vi "CSC_QuadPlannerLoose.vi"(5 "TorqueError(0)":T1, 6 "F range":cluster{"Fmin":dbl, "Fmax":dbl}, 7 "TargetF(N) (0)":dbl format="%#_13g", 8 "error in (no error)":errorcluster, 9 "LockedJoint":i32[](array[numeric]), 10 "DesireTorque(Nm)":dbl[](array[numeric]), 11 "C-Alex in":refnum<class "CableSerialChain.lvclass">) -> (0 "error out":errorcluster, 1 "Jacobian for Cables":T2, 2 "Planned Tension":dbl[](array[numeric]), 3 "C-Alex out":refnum<class "CableSerialChain.lvclass">, 4 "Solved":bool)   [LabVIEW 2015, in "CableSerialChain.lvclass"]
uses:
  CableSerialChain.lvclass
  <vilib>/Analysis/Matrix/Datatypes/RealMatrix.ctl
  <vilib>/gmath/NumericalOptimization/stopping criteria.ctl
  CableSerialChain.lvclass/CableSerialChain.ctl
  <vilib>/Analysis/7linalg.llb/Create Special Real Matrix.vi
  <vilib>/Analysis/Matrix/Numeric/Conversions/Matrix To Array - RM.vi
  <vilib>/gmath/NumericalOptimization/Quadratic Programming AS.vi
  <vilib>/gmath/NI_Gmath.lvlib
  <vilib>/Analysis/NI_AALPro.lvlib
  <vilib>/Analysis/Matrix/NI_Matrix.lvlib
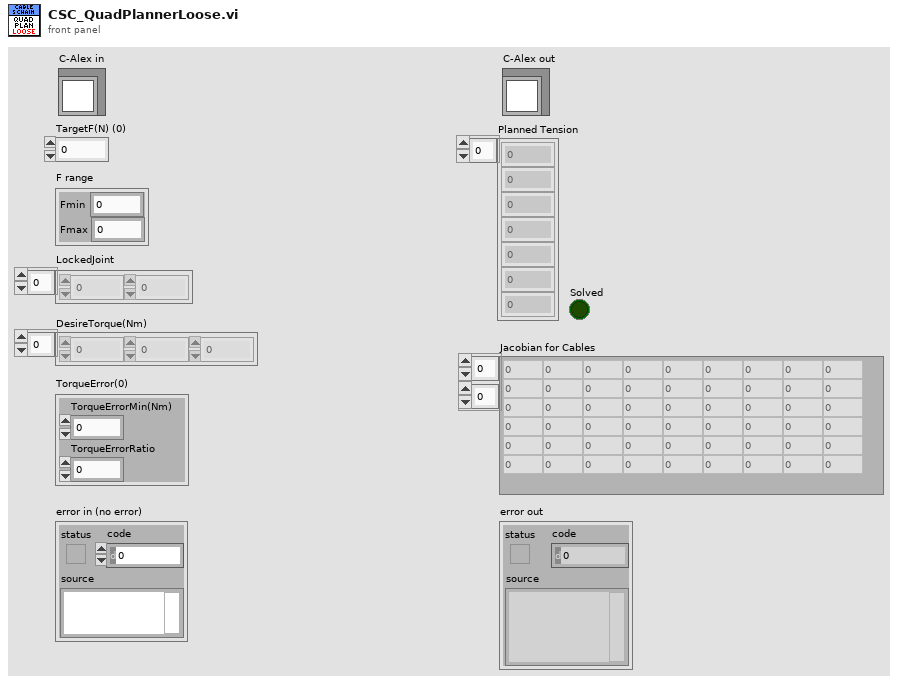
[diagram p1: front panel]
types:
  T1 = cluster{"TorqueErrorMin(Nm)":dbl, "TorqueErrorRatio":dbl}
  T2 = typedef "NI_Matrix.lvlib/RealMatrix.ctl" = dbl[][]
  T3 = typedef "NI_Gmath.lvlib/stopping criteria.ctl" = cluster{"function tolerance":dbl, "parameter tolerance":dbl, "max iterations":i32, "max function calls":i32, "gradient tolerance":dbl, "max time (sec)":dbl}
  T4 = typedef "CableSerialChain.lvclass/Cable.ctl" = cluster{"RoutingPtsInLCS":T5[], "Cable ID":i32, "ActiveSegments":i32[][]}
  T5 = typedef "Bodies.lvclass/PointOnBody.ctl" = cluster{"Coord4":dbl[], "ID":i32}
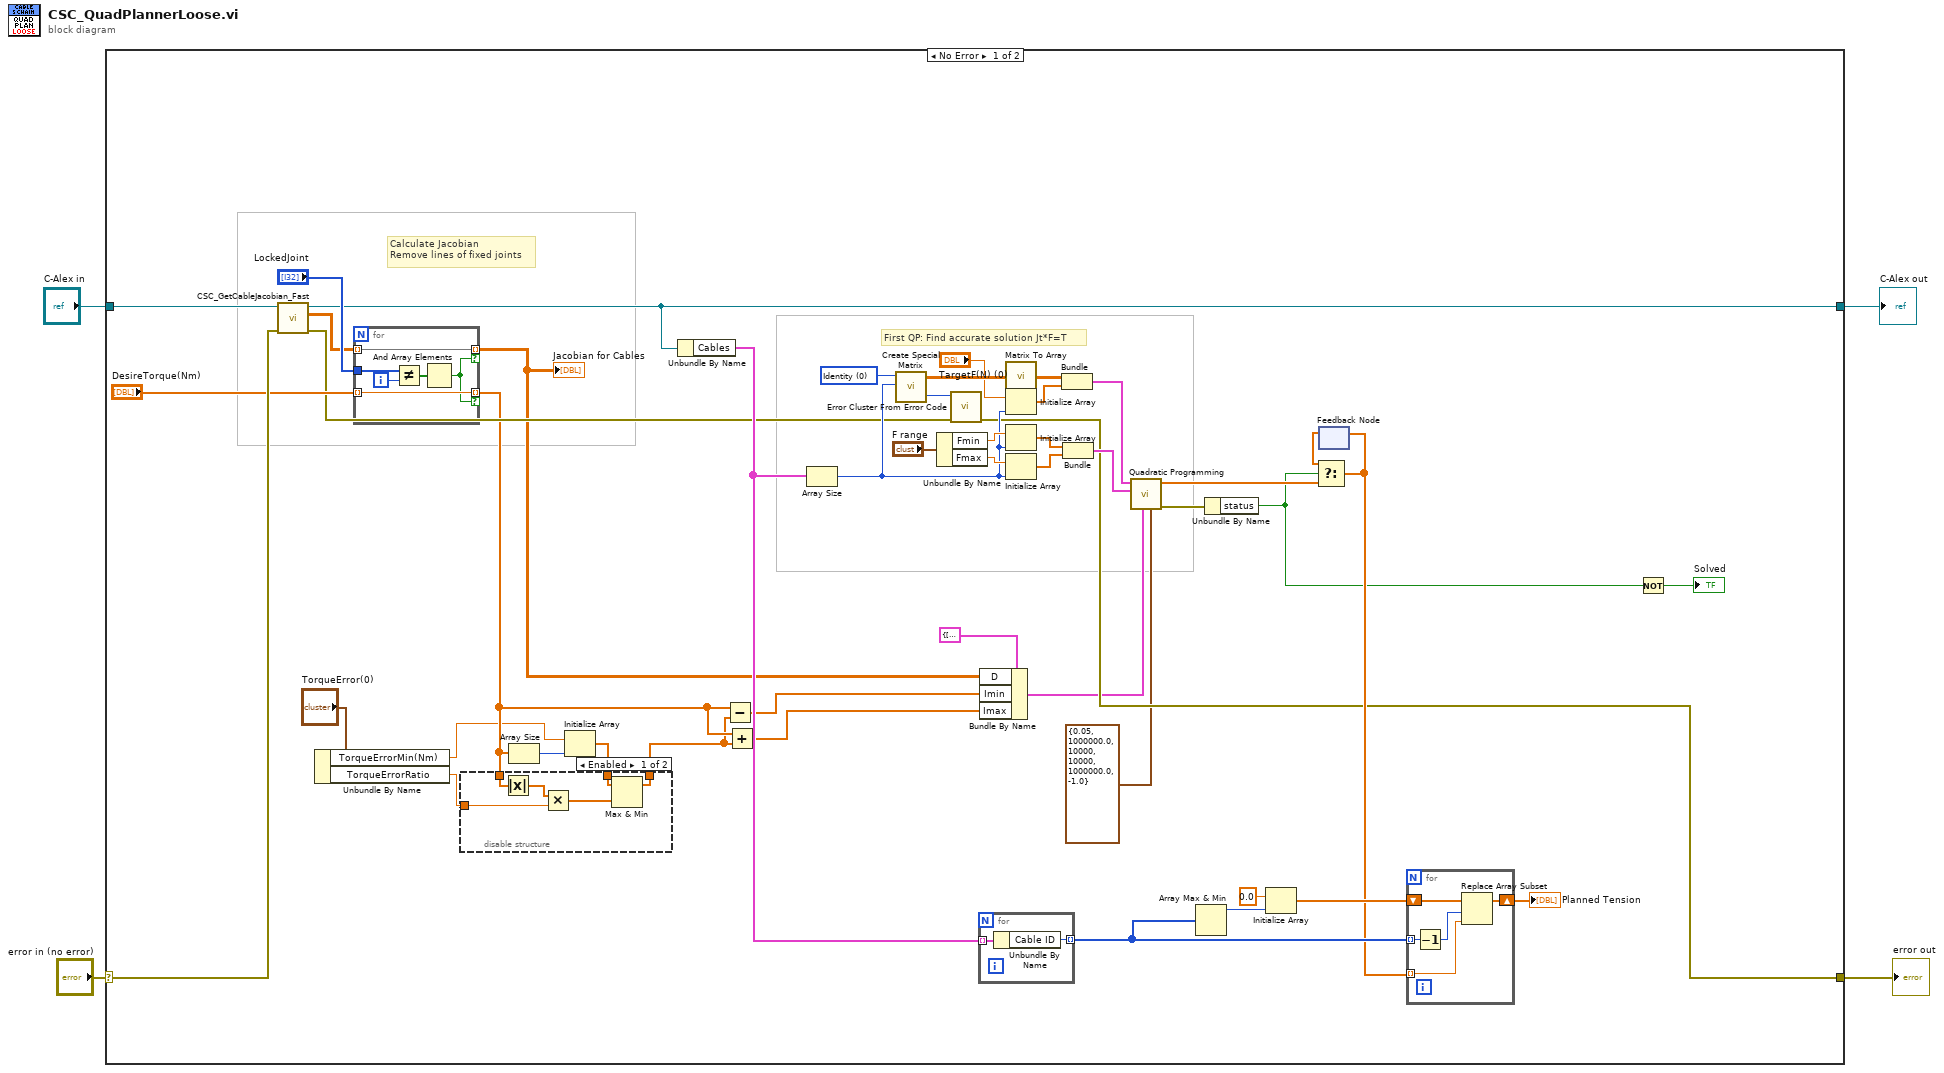
[diagram p0: block diagram]
diagram:
  n1 = case shown="No Error" "error in (no error)" {
    selector: "error in (no error)" -> [w28 w72]
    tunnel: [w22 w72] -> w3
    tunnel: [w26 w73] -> w1
    tunnel: "C-Alex in" -> [w30 w73]
    frame No Error {
      w46 = 0 items=["Identity", "Diagonal", "Toeplitz", "Vandermonde", "Companion", "Hankel", "Hadamard", "Wilkinson", "Hilbert", "Inverse Hilbert", "Rosser", "Pascal"] ("matrix type")
      # "First QP: Find accurate solution Jt*F=T"
      # "Calculate Jacobian\nRemove lines of fixed joints"
      n2 = call "CSC_GetCableJacobian_Fast.vi"("error in (no error)"=w28, "C-Alex in"=w30) -> ("error out"=w25:errorcluster, "Jacobian for Cables"=w36:T2, "C-Alex out"=w26:refnum<class "CableSerialChain.lvclass">)  [unwired: 7 in]
      n3 = Unbundle By Name("TorqueError(0)") -> ("TorqueErrorMin(Nm)"=w8:dbl, "TorqueErrorRatio"=w7:dbl)
      n4 = for {
        tunnel: "LockedJoint" -> [w70]
        tunnel: w36 -> [w68] mode=indexing
        tunnel: "DesireTorque(Nm)" -> [w67] mode=indexing
        tunnel: [w68] -> w13 mode=indexing if=w66
        tunnel: [w67] -> w12 mode=indexing if=w66
        i -> [w71]
        n5 = Not Equal?(x=w70, y=w71) -> (x != y?=w69:bool[])
        n6 = And Array Elements(Boolean array=w69) -> (logical AND=w66:bool)
      }
      "Jacobian for Cables" <- w13
      n7 = Array Size(array=w12) -> (size(s)=w18:i32)
      n8 = Initialize Array(w8, w18) -> (w11:dbl[])
      n9 = disable-structure shown="Enabled" {
        disable-tunnel: w12 -> [w57 _]
        disable-tunnel: w11 -> [w55 w58]
        disable-tunnel: [w53 w58] -> w10
        disable-tunnel: w7 -> [w52 _]
        frame Enabled {
          n10 = Absolute Value(x=w57) -> (abs(x)=w56:dbl[])
          n11 = Multiply(x=w56, y=w52) -> (x*y=w54:dbl[])
          n12 = Max & Min(x=w55, y=w54) -> (max(x,y)=w53:dbl[])  [unwired: 1 out]
        }
        frame Disabled {
        }
      }
      n13 = Unbundle By Name(w26) -> ("Cables"=w29:T4[])
      n14 = Subtract(x=w12, y=w10) -> (x-y=w17:dbl[])
      n15 = Add(x=w12, y=w10) -> (x+y=w16:dbl[])
      n16 = Array Size(array=w29) -> (size(s)=w39:i32)
      n17 = call-poly <vilib>:"Create Special Matrix.vi"("matrix type"=w46, "matrix size"=w39) -> ("Special Matrix"=w45:T2, "error"=w42:i32)  [unwired: 3 in]
      n18 = Unbundle By Name("F range") -> ("Fmin"=w50:dbl, "Fmax"=w49:dbl)
      n19 = call <vilib>:"Error Cluster From Error Code.vi"("error in (no error)"=w25, "error code (0)"=w42) -> ("error out"=w22:errorcluster)  [unwired: 7 in]
      n20 = for {
        tunnel: w29 -> [w65] mode=indexing
        tunnel: [w64] -> w34 mode=indexing
        n21 = Unbundle By Name(w65) -> ("Cable ID"=w64:i32)
      }
      n22 = Bundle By Name(cluster=cluster{"D":dbl[][], "Imin":dbl[], "Imax":dbl[]} {"D"=[], "Imin"=[], "Imax"=[]} ("inequality constraints"), "D"=w13, "Imin"=w17, "Imax"=w16) -> (w19:cluster{"D":dbl[][], "Imin":dbl[], "Imax":dbl[]})
      n23 = call-poly <vilib>:"Matrix To Array.vi"("Real Matrix"=w45) -> ("Real 2D Array"=w44:dbl[][])
      n24 = Initialize Array("TargetF(N) (0)", w39) -> (w37:dbl[])
      n25 = Initialize Array(w50, w39) -> (w41:dbl[])
      n26 = Initialize Array(w49, w39) -> (w48:dbl[])
      n27 = Bundle("Real 2D Array"=w44, w37) -> (w43:cluster{"Real 2D Array":dbl[][], dbl[]})  [unwired: 1 in]
      n28 = Bundle(w41, w48) -> (w47:cluster{dbl[], dbl[]})  [unwired: 1 in]
      n29 = call-poly <vilib>:"Quadratic Programming.vi"("stopping criteria"=T3 {"function tolerance"=0.05, "parameter tolerance"=1000000.0, "max iterations"=10000, "max function calls"=10000, "gradient tolerance"=1000000.0, "max time (sec)"=-1.0}, "inequality constraints"=w19, "parameter bounds"=w47, "objective function"=w43) -> ("error out"=w21:errorcluster, "minimum"=w24:dbl[])  [unwired: 4 in, 2 out]
      n30 = Array Max & Min(array=w34) -> (max value=w33:i32)  [unwired: 3 out]
      n31 = Unbundle By Name(w21) -> ("status"=w15:bool)
      n32 = Initialize Array(0.0 ("element"), w33) -> (w32:dbl[])
      n33 = feedback #1() -> (w5:dbl[])  [unwired: 1 in]
      n34 = Select(t=w5, s=w15, f=w24) -> (s? t:f=w23:dbl[])
      n35 = feedback-in #1(w23) -> ()
      n36 = for {
        tunnel: w34 -> [w63] mode=indexing
        shift-right: [w61] -> w14
        shift-left: w32 -> [w60]
        tunnel: w23 -> [w59] mode=indexing
        n37 = Decrement(x=w63) -> (x-1=w62:i32)
        n38 = Replace Array Subset(array=w60, new element=w59, index=w62) -> (w61:dbl[])
      }
      "Planned Tension" <- w14
      n39 = Not(x=w15) -> (.not. x?=→"Solved":bool)
    }
    frame Error {
    }
  }
  "error out" <- w3
  "C-Alex out" <- w1
